vi "RampSetup.vi"() -> ()   [LabVIEW 2009]
doc: "Einstellungen für die Betriebsart \"Intensitäts-Rampe\"."
panel:
  in  "RampSetting":T1={"use"=FALSE, "steps"=2, "start (V)"=0.0, "stop (V)"=0.0, "periode (s)"=30.0, "manual"=[]} {"periode (s)" min=0.001; "stop (V)" min=0.0 max=10.0; "start (V)" min=0.0 max=10.0; "steps" min=1 step=1}
  in  "Cancel":bool
  in  "OK":bool
  # "voltage (V)"
  # "time (s)"
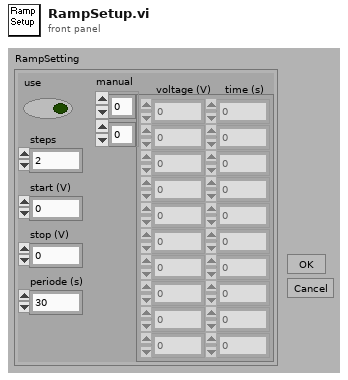
[diagram p1: front panel]
types:
  T1 = cluster{"use":bool, "steps":u16, "start (V)":dbl, "stop (V)":dbl, "periode (s)":dbl, "manual":dbl[][]}
  T2 = cluster{"used":bool, "steps":u16, "start (V)":dbl, "stop (V)":dbl, "periode (s)":dbl, dbl[][]}
  T3 = cluster{"used":bool, "steps":u16, "start (V)":dbl, "stop (V)":dbl, "periode (s)":dbl, "manual":dbl[][]}
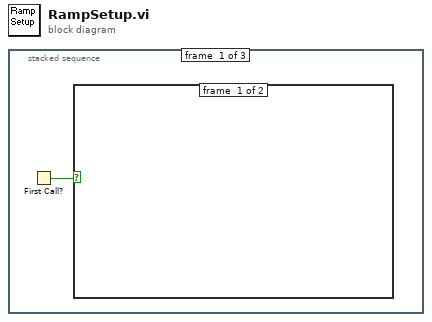
[diagram p0: block diagram]
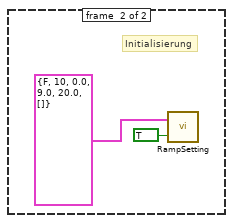
[diagram p2: hidden frame]
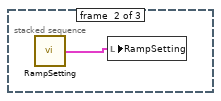
[diagram p3: hidden frame]
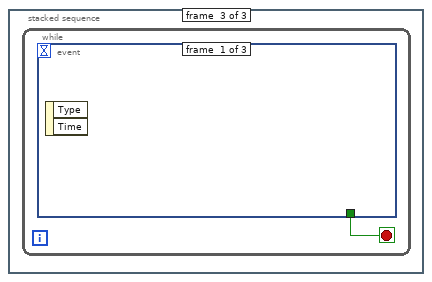
[diagram p4: hidden frame]
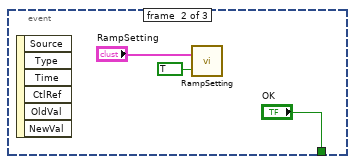
[diagram p5: hidden frame]
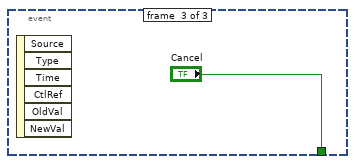
[diagram p6: hidden frame]
diagram:
  n1 = stacked-sequence {
    frame #0 {
      n2 = First Call?() -> (First Call?: T/F=w1:bool)
      n3 = case shown="True" w1 {
        frame #0 {
        }
        frame #1 {
          # "Initialisierung"
          n4 = call "RampSetting.vi"("set/get"=TRUE, "RampSetting (in)"=T2 {"used"=FALSE, "steps"=10, "start (V)"=0.0, "stop (V)"=9.0, "periode (s)"=20.0, []}) -> ()  [unwired: 1 out]
        }
      }
    }
    frame #1 {
      n5 = call "RampSetting.vi"() -> ("RampSetting (out)"=w4:T3)  [unwired: 2 in]
      n6 = local write "RampSetting"(w4) -> ()
    }
    frame #2 {
      n7 = while {
        stop <- w5 stop-if-true
        n8 = event shown="[1] \"OK\": Value Change" {
          selector: _ -> [_ _ _]
          dyn-events: _ -> [_ _ _]
          timeout: _ -> [_ _ _]
          tunnel: [_ "OK" "Cancel"] -> w5
          event #0 {
            n9 = event-data() -> ()  [unwired: 1 in, 2 out]
          }
          event #1 {
            n10 = event-data() -> ()  [unwired: 1 in, 6 out]
            n11 = call "RampSetting.vi"("set/get"=TRUE, "RampSetting (in)"="RampSetting") -> ()  [unwired: 1 out]
          }
          event #2 {
            n12 = event-data() -> ()  [unwired: 1 in, 6 out]
          }
        }
      }
    }
  }
